vi "physical mapping.vi"() -> ()   [LabVIEW 2015]
uses:
  <vilib>/Utility/file.llb/Read Delimited Spreadsheet (I64).vi
panel:
  out "Intensity Graph":i32[][](graph)
  out "Intensity Graph 2":i32[][](graph)
  out "Intensity Graph 3":i32[][](graph)
  out "Intensity Graph 4":i32[][](graph)
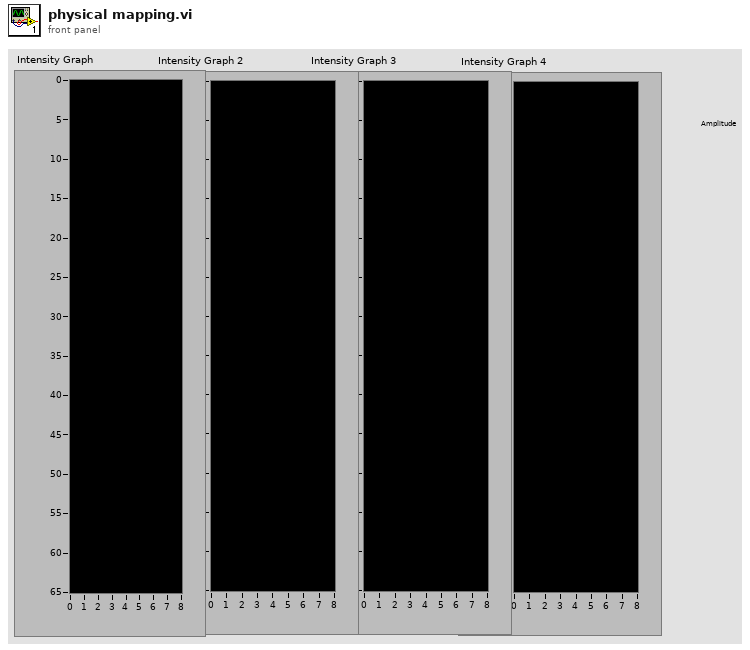
[diagram p1: front panel]
types:
  T1 = typedef "imagedata.ctl" = cluster{"image type":i32, "image depth":i32, "image":u8[], "mask":u8[], "colors":u32[], "Rectangle":cluster{"left":i16, "top":i16, "right":i16, "bottom":i16}}
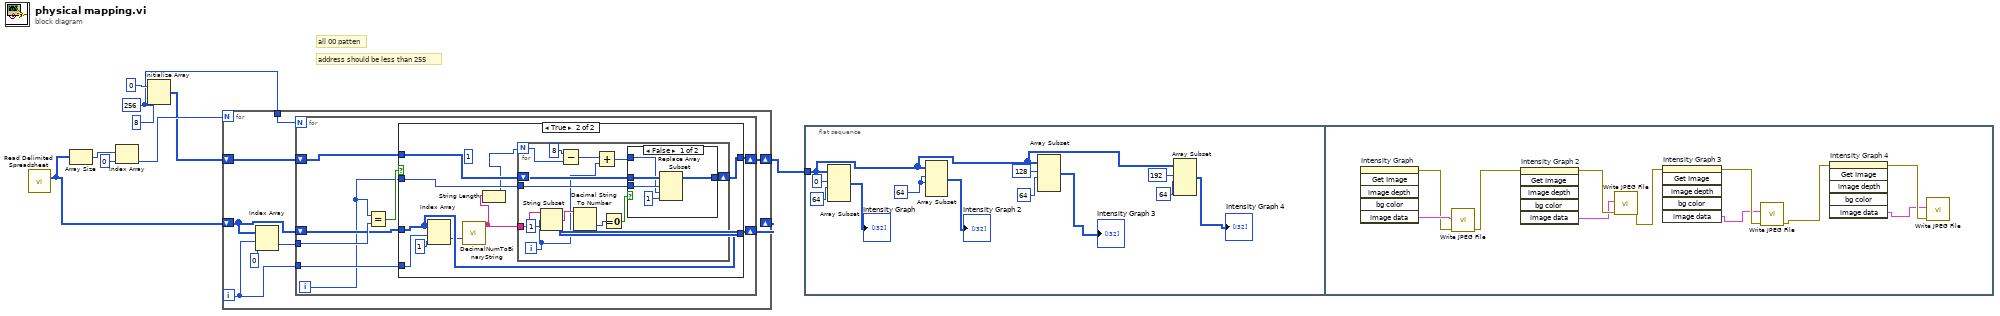
[diagram p0: block diagram]
diagram:
  w2 = 256 ("维数大小")
  # "address should be less than 255"
  # "all 00 patten"
  n1 = call-poly <vilib>:"Read Delimited Spreadsheet.vi"() -> ("all rows"=w3:i64[][])  [unwired: 10 in, 5 out]
  n2 = Array Size(array=w3) -> (size(s)=w7:i32[])
  n3 = Index Array(array=w7, index=0 ("索引")) -> (element=w5:i32)
  n4 = Initialize Array(0, w2, 8 ("dimension size")) -> (w4:i32[][])
  n5 = for {
    N: w5 -> [_]
    shift-right: [w11] -> _
    shift-left: w3 -> [w14]
    shift-right: [w12] -> w1
    shift-left: w4 -> [w16]
    tunnel: w2 -> [w10]
    i -> [w13]
    n6 = Index Array(array=w14, index (row)=w13, index (col)=0 ("禁用的索引 (列)")) -> (element=w15:i64)
    n7 = for {
      N: w10 -> [_]
      shift-right: [w20] -> w12
      shift-left: w16 -> [w25]
      tunnel: w15 -> [w24]
      shift-right: [w19] -> w11
      shift-left: w14 -> [w22]
      tunnel: w13 -> [w21]
      i -> [w18]
      n8 = Equal?(x=w18, y=w24) -> (x = y?=w23:bool)
      n9 = case shown="True" w23 {
        tunnel: w25 -> [w27 w33]
        tunnel: w18 -> [_ w32]
        tunnel: w22 -> [w26 w30]
        tunnel: w21 -> [_ w36]
        tunnel: [w27 w31] -> w20
        tunnel: [w26 w30] -> w19
        frame False {
        }
        frame True {
          (unwired) i64 1 ("y")
          n10 = Index Array(array=w30, index (row)=w36, index (col)=1 ("禁用的索引 (列)")) -> (element=w29:i64)
          n11 = call "DecimalNumToBinaryString.vi"("十进制 整形"=w29) -> ("二进制字符串"=w34:string)  [unwired: 10 in]
          n12 = String Length(string=w34) -> (length=w28:i32)
          n13 = for {
            N: w28 -> [w43]
            tunnel: w34 -> [w49]
            tunnel: w32 -> [w44]
            shift-right: [w41] -> w31
            shift-left: w33 -> [w45]
            i -> [w37]
            n14 = String Subset(string=w49, offset (0)=w37, length (rest)=1 ("长度（剩余）")) -> (substring=w47:string)
            n15 = Subtract(x=8, y=w43) -> (x-y=w38:i32)
            n16 = Decimal String To Number(string=w47) -> (number=w40:i32)  [unwired: 2 in, 1 out]
            n17 = Add(x=w38, y=w37) -> (x+y=w39:i32)
            n18 = Equal To 0?(x=w40) -> (x = 0?=w46:bool)
            n19 = case shown="False" w46 {
              tunnel: w45 -> [w54 w55]
              tunnel: w44 -> [w53 _]
              tunnel: w39 -> [w52 _]
              tunnel: [w50 w55] -> w41
              frame False {
                n20 = Replace Array Subset(array=w54, new element=1 ("新元素/子数组"), index (row)=w53, index (col)=w52) -> (w50:i32[][])
              }
              frame True {
              }
            }
          }
        }
      }
    }
  }
  n21 = flat-sequence {
    tunnel: w1 -> [w59]
    frame #0 {
      w63 = 64 ("长度")
      n22 = Array Subset(array=w59, index (row)=0 ("索引"), length (row)=64 ("长度")) -> (→"Intensity Graph":i32[][])  [unwired: 2 in]
      n23 = Array Subset(array=w59, index (row)=w63, length (row)=w63) -> (→"Intensity Graph 2":i32[][])  [unwired: 2 in]
      n24 = Array Subset(array=w59, index (row)=128 ("索引"), length (row)=64 ("长度")) -> (→"Intensity Graph 3":i32[][])  [unwired: 2 in]
      n25 = Array Subset(array=w59, index (row)=192 ("索引"), length (row)=64 ("长度")) -> (→"Intensity Graph 4":i32[][])  [unwired: 2 in]
    }
    frame #1 {
      n26 = invoke on="Intensity Graph" class="IntGraph (严格)" method="Get Image"() -> (error out=w71:errorcluster, "image data"=w72:T1)  [unwired: 6 in, 4 out]
      n27 = call <vilib>:"Write JPEG File.vi"("error in (no error)"=w71, "image data"=w72) -> ("error out"=w77:errorcluster)  [unwired: 8 in, 1 out]
      n28 = invoke on="Intensity Graph 2" class="IntGraph (严格)" method="Get Image"(error in=w77) -> (error out=w74:errorcluster, "image data"=w73:T1)  [unwired: 5 in, 4 out]
      n29 = call <vilib>:"Write JPEG File.vi"("error in (no error)"=w74, "image data"=w73) -> ("error out"=w78:errorcluster)  [unwired: 8 in, 1 out]
      n30 = invoke on="Intensity Graph 3" class="IntGraph (严格)" method="Get Image"(error in=w78) -> (error out=w76:errorcluster, "image data"=w75:T1)  [unwired: 5 in, 4 out]
      n31 = call <vilib>:"Write JPEG File.vi"("error in (no error)"=w76, "image data"=w75) -> ("error out"=w68:errorcluster)  [unwired: 8 in, 1 out]
      n32 = invoke on="Intensity Graph 4" class="IntGraph (严格)" method="Get Image"(error in=w68) -> (error out=w70:errorcluster, "image data"=w69:T1)  [unwired: 5 in, 4 out]
      n33 = call <vilib>:"Write JPEG File.vi"("error in (no error)"=w70, "image data"=w69) -> ()  [unwired: 8 in, 2 out]
    }
  }
